vi "Cluster67ToCluster8.vi"(0 "Cluster67":T4) -> (2 "Cluster8":T1)   [LabVIEW 2019]
uses:
  Cluster67.ctl
  Test_data.ctl
  Test_load.ctl
  Hardness_test.ctl
  TEST.lvclass
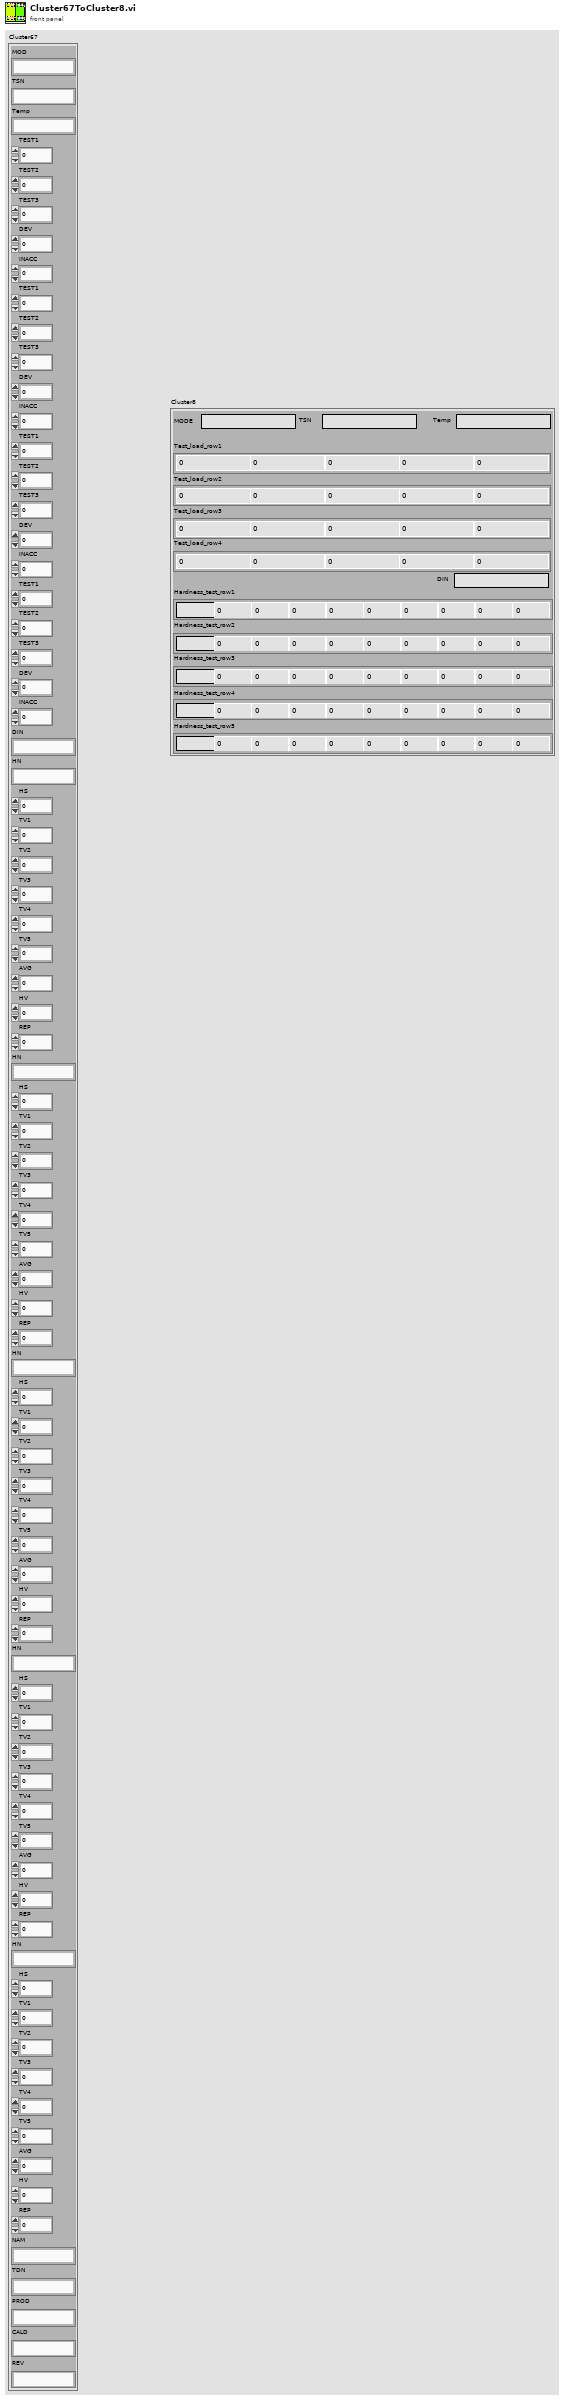
[diagram p1: front panel]
types:
  T1 = typedef "TEST.lvclass/Test_data.ctl" = cluster{"MODE":string, "TSN":string, "Temp":string, "Test_load_row1":T2, "Test_load_row2":T2, "Test_load_row3":T2, "Test_load_row4":T2, "DIN":string, "Hardness_test_row1":T3, "Hardness_test_row2":T3, "Hardness_test_row3":T3, "Hardness_test_row4":T3, "Hardness_test_row5":T3}
  T2 = typedef "TEST.lvclass/Test_load.ctl" = cluster{"TEST1":sgl, "TEST2":sgl, "TEST3":sgl, "DEV":sgl, "INACC":sgl}
  T3 = typedef "TEST.lvclass/Hardness_test.ctl" = cluster{"HN":string, "HS":sgl, "TV1":sgl, "TV2":sgl, "TV3":sgl, "TV4":sgl, "TV5":sgl, "AVG":sgl, "HV":sgl, "REP":sgl}
  T4 = typedef "TEST.lvclass/Cluster67.ctl" = cluster{"MOD":string, "TSN":string, "Temp":string, "TEST1":sgl, "TEST2":sgl, "TEST3":sgl, "DEV":sgl, "INACC":sgl, "TEST1":sgl, "TEST2":sgl, "TEST3":sgl, "DEV":sgl, "INACC":sgl, "TEST1":sgl, "TEST2":sgl, "TEST3":sgl, "DEV":sgl, "INACC":sgl, "TEST1":sgl, "TEST2":sgl, "TEST3":sgl, "DEV":sgl, "INACC":sgl, "DIN":string, "HN":string, "HS":sgl, "TV1":sgl, "TV2":sgl, "TV3":sgl, "TV4":sgl, "TV5":sgl, "AVG":sgl, "HV":sgl, "REP":sgl, "HN":string, "HS":sgl, "TV1":sgl, "TV2":sgl, "TV3":sgl, "TV4":sgl, "TV5":sgl, "AVG":sgl, "HV":sgl, "REP":sgl, "HN":string, "HS":sgl, "TV1":sgl, "TV2":sgl, "TV3":sgl, "TV4":sgl, "TV5":sgl, "AVG":sgl, "HV":sgl, "REP":sgl, "HN":string, "HS":sgl, "TV1":sgl, "TV2":sgl, "TV3":sgl, "TV4":sgl, "TV5":sgl, "AVG":sgl, "HV":sgl, "REP":sgl, "HN":string, "HS":sgl, "TV1":sgl, "TV2":sgl, "TV3":sgl, "TV4":sgl, "TV5":sgl, "AVG":sgl, "HV":sgl, "REP":sgl, "NAM":string, "TDN":string, "PROD":string, "CALD":string, "REV":string}
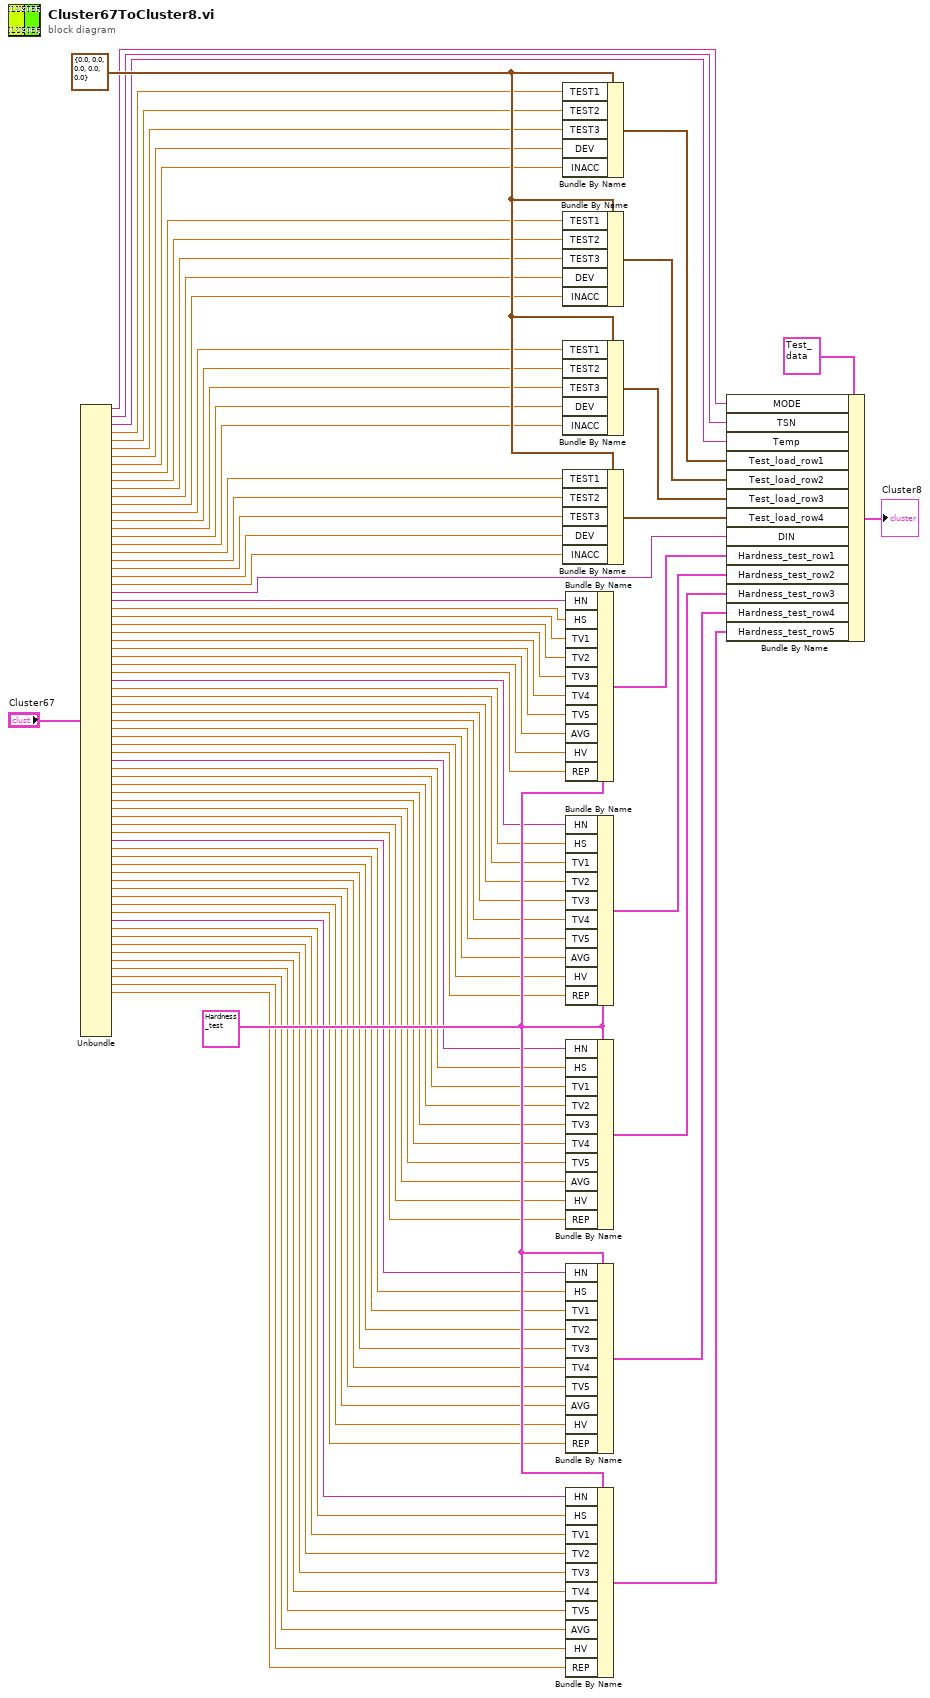
[diagram p0: block diagram]
diagram:
  w87 = T3 {"HN"="", "HS"=0.0, "TV1"=0.0, "TV2"=0.0, "TV3"=0.0, "TV4"=0.0, "TV5"=0.0, "AVG"=0.0, "HV"=0.0, "REP"=0.0} ("Hardness_test")
  w81 = T2 {"TEST1"=0.0, "TEST2"=0.0, "TEST3"=0.0, "DEV"=0.0, "INACC"=0.0} ("Test_load")
  n1 = Unbundle("Cluster67") -> ("MOD"=w72:string, "TSN"=w74:string, "Temp"=w73:string, "TEST1"=w71:sgl, "TEST2"=w70:sgl, "TEST3"=w69:sgl, "DEV"=w68:sgl, "INACC"=w67:sgl, "TEST1"=w66:sgl, "TEST2"=w65:sgl, "TEST3"=w61:sgl, "DEV"=w60:sgl, "INACC"=w59:sgl, "TEST1"=w58:sgl, "TEST2"=w57:sgl, "TEST3"=w56:sgl, "DEV"=w55:sgl, "INACC"=w54:sgl, "TEST1"=w53:sgl, "TEST2"=w52:sgl, "TEST3"=w51:sgl, "DEV"=w50:sgl, "INACC"=w49:sgl, "DIN"=w64:string, "HN"=w63:string, "HS"=w48:sgl, "TV1"=w47:sgl, "TV2"=w46:sgl, "TV3"=w45:sgl, "TV4"=w44:sgl, "TV5"=w43:sgl, "AVG"=w42:sgl, "HV"=w41:sgl, "REP"=w40:sgl, "HN"=w62:string, "HS"=w39:sgl, "TV1"=w38:sgl, "TV2"=w37:sgl, "TV3"=w36:sgl, "TV4"=w35:sgl, "TV5"=w34:sgl, "AVG"=w33:sgl, "HV"=w32:sgl, "REP"=w31:sgl, "HN"=w30:string, "HS"=w29:sgl, "TV1"=w28:sgl, "TV2"=w27:sgl, "TV3"=w26:sgl, "TV4"=w25:sgl, "TV5"=w24:sgl, "AVG"=w23:sgl, "HV"=w22:sgl, "REP"=w21:sgl, "HN"=w20:string, "HS"=w19:sgl, "TV1"=w18:sgl, "TV2"=w17:sgl, "TV3"=w16:sgl, "TV4"=w15:sgl, "TV5"=w14:sgl, "AVG"=w13:sgl, "HV"=w12:sgl, "REP"=w11:sgl, "HN"=w10:string, "HS"=w9:sgl, "TV1"=w8:sgl, "TV2"=w7:sgl, "TV3"=w6:sgl, "TV4"=w5:sgl, "TV5"=w4:sgl, "AVG"=w3:sgl, "HV"=w2:sgl, "REP"=w1:sgl)  [unwired: 5 out]
  n2 = Bundle By Name(cluster=w81, "TEST1"=w71, "TEST2"=w70, "TEST3"=w69, "DEV"=w68, "INACC"=w67) -> (w85:T2)
  n3 = Bundle By Name(cluster=w81, "TEST1"=w66, "TEST2"=w65, "TEST3"=w61, "DEV"=w60, "INACC"=w59) -> (w84:T2)
  n4 = Bundle By Name(cluster=w81, "TEST1"=w58, "TEST2"=w57, "TEST3"=w56, "DEV"=w55, "INACC"=w54) -> (w83:T2)
  n5 = Bundle By Name(cluster=w81, "TEST1"=w53, "TEST2"=w52, "TEST3"=w51, "DEV"=w50, "INACC"=w49) -> (w80:T2)
  n6 = Bundle By Name(cluster=w87, "HN"=w63, "HS"=w48, "TV1"=w47, "TV2"=w46, "TV3"=w45, "TV4"=w44, "TV5"=w43, "AVG"=w42, "HV"=w41, "REP"=w40) -> (w79:T3)
  n7 = Bundle By Name(cluster=w87, "HN"=w62, "HS"=w39, "TV1"=w38, "TV2"=w37, "TV3"=w36, "TV4"=w35, "TV5"=w34, "AVG"=w33, "HV"=w32, "REP"=w31) -> (w78:T3)
  n8 = Bundle By Name(cluster=w87, "HN"=w30, "HS"=w29, "TV1"=w28, "TV2"=w27, "TV3"=w26, "TV4"=w25, "TV5"=w24, "AVG"=w23, "HV"=w22, "REP"=w21) -> (w77:T3)
  n9 = Bundle By Name(cluster=w87, "HN"=w20, "HS"=w19, "TV1"=w18, "TV2"=w17, "TV3"=w16, "TV4"=w15, "TV5"=w14, "AVG"=w13, "HV"=w12, "REP"=w11) -> (w76:T3)
  n10 = Bundle By Name(cluster=w87, "HN"=w10, "HS"=w9, "TV1"=w8, "TV2"=w7, "TV3"=w6, "TV4"=w5, "TV5"=w4, "AVG"=w3, "HV"=w2, "REP"=w1) -> (w75:T3)
  n11 = Bundle By Name(cluster=T1 {"MODE"="", "TSN"="", "Temp"="", "Test_load_row1"={"TEST1"=0.0, "TEST2"=0.0, "TEST3"=0.0, "DEV"=0.0, "INACC"=0.0}, "Test_load_row2"={"TEST1"=0.0, "TEST2"=0.0, "TEST3"=0.0, "DEV"=0.0, "INACC"=0.0}, "Test_load_row3"={"TEST1"=0.0, "TEST2"=0.0, "TEST3"=0.0, "DEV"=0.0, "INACC"=0.0}, "Test_load_row4"={"TEST1"=0.0, "TEST2"=0.0, "TEST3"=0.0, "DEV"=0.0, "INACC"=0.0}, "DIN"="", "Hardness_test_row1"={"HN"="", "HS"=0.0, "TV1"=0.0, "TV2"=0.0, "TV3"=0.0, "TV4"=0.0, "TV5"=0.0, "AVG"=0.0, "HV"=0.0, "REP"=0.0}, "Hardness_test_row2"={"HN"="", "HS"=0.0, "TV1"=0.0, "TV2"=0.0, "TV3"=0.0, "TV4"=0.0, "TV5"=0.0, "AVG"=0.0, "HV"=0.0, "REP"=0.0}, "Hardness_test_row3"={"HN"="", "HS"=0.0, "TV1"=0.0, "TV2"=0.0, "TV3"=0.0, "TV4"=0.0, "TV5"=0.0, "AVG"=0.0, "HV"=0.0, "REP"=0.0}, "Hardness_test_row4"={"HN"="", "HS"=0.0, "TV1"=0.0, "TV2"=0.0, "TV3"=0.0, "TV4"=0.0, "TV5"=0.0, "AVG"=0.0, "HV"=0.0, "REP"=0.0}, "Hardness_test_row5"={"HN"="", "HS"=0.0, "TV1"=0.0, "TV2"=0.0, "TV3"=0.0, "TV4"=0.0, "TV5"=0.0, "AVG"=0.0, "HV"=0.0, "REP"=0.0}} ("簇"), "MODE"=w72, "TSN"=w74, "Temp"=w73, "Test_load_row1"=w85, "Test_load_row2"=w84, "Test_load_row3"=w83, "Test_load_row4"=w80, "DIN"=w64, "Hardness_test_row1"=w79, "Hardness_test_row2"=w78, "Hardness_test_row3"=w77, "Hardness_test_row4"=w76, "Hardness_test_row5"=w75) -> (→"Cluster8":T1)
